vi "Result.Measurement Status to String, for XLink.vi"(4 "Fail = OutOfTolerance":bool, 7 "Status":T1 items=["LOG", "PASS", "FAIL", "ERROR"]) -> (2 "resulting string":string)   [LabVIEW 2019]
uses:
  Result.Measurement and Attribute Item Status.ctl
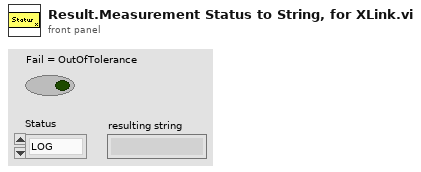
[diagram p1: front panel]
types:
  T1 = typedef "Result.Measurement and Attribute Item Status.ctl" = i32
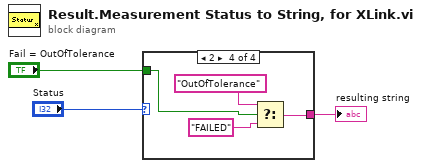
[diagram p0: block diagram]
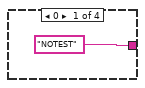
[diagram p2: hidden frame]
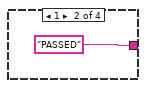
[diagram p3: hidden frame]
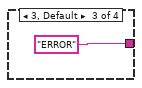
[diagram p4: hidden frame]
diagram:
  n1 = case shown="2" "Status" {
    tunnel: ["NOTEST" "PASSED" "ERROR" w10] -> w2
    tunnel: "Fail = OutOfTolerance" -> [_ _ _ w7]
    frame 0 {
    }
    frame 1 {
    }
    frame 3, Default {
    }
    frame 2 {
      n2 = Select(t="OutOfTolerance", s=w7, f="FAILED") -> (s? t:f=w10:string)
    }
  }
  "resulting string" <- w2
